vi "trash_Update Clock Map Command.vi"(8 "error in":errorcluster, 10 "Clock Conversion":T1, 11 "CoreOOB_Rx in":refnum<class "ChanMngOOB_Rx.lvclass">) -> (0 "error out":errorcluster, 3 "CoreOOB_Rx out":refnum<class "ChanMngOOB_Rx.lvclass">)   [LabVIEW 2021]
uses:
  ChanMngOOB_Rx.lvclass/ChanMngOOB_Rx.ctl
  <vilib>/CIF Foundation/CIF Out of Band Commands/CIFOutOfBand.lvclass
  Typedef/OOB ChnMng Commands.ctl
  ChanMngOOB_Rx.lvclass
  Typedef/Template Payload.ctl
  Typedef/Channel Connection Data.ctl
  Typedef/Channel Fault Data.ctl
  <vilib>/CIF Foundation/CIF Out of Band Commands/Typedef/OOB Container.ctl
  C:/Program Files/National Instruments/LabVIEW 2021/vi.lib/CIF Foundation/CIF Out of Band Commands/CIFOutOfBand.lvclass
  <vilib>/CIF Foundation/CIF Utilities/Time/Typedef/Timestamp Pair.ctl
  <vilib>/CIF Foundation/CIF Utilities/Time/Time_CIF_U.lvlib
  <vilib>/CIF Foundation/CIF Utilities/Time/Typedef/Clock Conversion Map.ctl
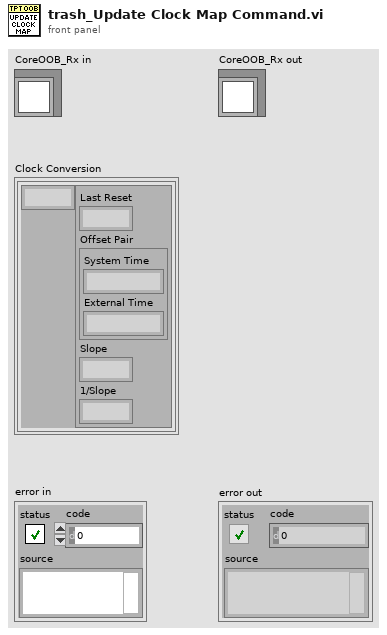
[diagram p1: front panel]
types:
  T1 = typedef "Time_CIF_U.lvlib/Clock Conversion Map.ctl" = map{u8, cluster{"Last Reset":i64, "Offset Pair":T2, "Slope":dbl, "1/Slope":dbl}}
  T2 = typedef "Time_CIF_U.lvlib/Timestamp Pair.ctl" = cluster{"System Time":i64, "External Time":i64}
  T3 = typedef "CIFOutOfBand.lvclass/OOB Container.ctl" = cluster{"Commands (bitwise)":u64, "Payload":variant}
  T4 = typedef "ChanMngOOB_Rx.lvclass/OOB ChnMng Commands.ctl" = enum8{"Start", "Pause", "Stop", "RefreshStats", "UpdateConfig", "Connect Channel", "Force Channel", "Update Clock Map"}
  T5 = typedef "ChanMngOOB_Rx.lvclass/Template Payload.ctl" = cluster{"Connections":T6[], "Forces":T7[]}
  T6 = typedef "ChanMngOOB_Rx.lvclass/Channel Connection Data.ctl" = cluster{"Publisher Name":string, "Subscriber Name":string, "Connection Data":u8[]}
  T7 = typedef "ChanMngOOB_Rx.lvclass/Channel Fault Data.ctl" = cluster{"Channel Name":string, "Force Data":u8[], "Force Active":bool}
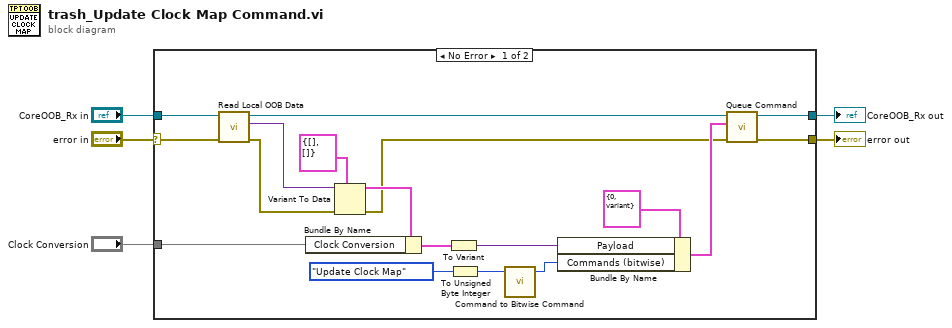
[diagram p0: block diagram]
diagram:
  n1 = case shown="No Error" "error in" {
    selector: "error in" -> [w20 w25]
    tunnel: [w22 w25] -> w4
    tunnel: "CoreOOB_Rx in" -> [w21 w24]
    tunnel: [w23 w24] -> w2
    tunnel: "Clock Conversion" -> [w12 _]
    frame No Error {
      n2 = call <vilib>:"Read Local OOB Data.vi"("error in"=w20, "OOB in"=w21) -> ("error out"=w16:errorcluster, "Local OOB Data"=w19:variant, "OOB out"=w6:refnum<class "ChanMngOOB_Rx.lvclass">)  [unwired: 7 in]
      n3 = Variant To Data(error in=w16, type=T5 {"Connections"=[], "Forces"=[]} ("Template Payload"), Variant=w19) -> (data=w17:T5, error out=w7:errorcluster)
      n4 = Bundle By Name(cluster=w17, "Clock Conversion"=w12) -> (w13:T5)
      n5 = To Variant(anything=w13) -> (Variant=w10:variant)
      n6 = To Unsigned Byte Integer(number=OOB_ChnMng_Commands."Update Clock Map" ("OOB Main Commands")) -> (unsigned 8bit integer=w15:u8)
      n7 = call <vilib>:"Command to Bitwise Command.vi"("Command"=w15) -> ("bit command"=w9:u64)  [unwired: 3 in]
      n8 = Bundle By Name(cluster=T3 {"Commands (bitwise)"=0, "Payload"=variant} ("OOB Data"), "Payload"=w10, "Commands (bitwise)"=w9) -> (w8:T3)
      n9 = call <vilib>:"Queue Command.vi"("error in"=w7, "OOB Data"=w8, "OOB in"=w6) -> ("error out"=w22:errorcluster, "OOB out"=w23:refnum<class "ChanMngOOB_Rx.lvclass">)  [unwired: 7 in]
    }
    frame Error {
    }
  }
  "error out" <- w4
  "CoreOOB_Rx out" <- w2
